vi "Configure Fixed Ref Junction [TC] Core.vi"(8 "error in (no error)":errorcluster, 10 "fixed ref junc (0.0 Celsius)":dbl format="%^.2e", 11 "IVI_DMM in":refnum<class "IVI_DMM.lvclass">) -> (0 "error out":errorcluster, 3 "IVI_DMM out":refnum<class "IVI_DMM.lvclass">)   [LabVIEW 2013, in "IVI_DMM.lvlib" / "IVI_DMM.lvclass"]
doc: "This VI configures the fixed reference junction for a thermocouple with a fixed reference junction type.\n\nThis VI affects the behavior of the instrument only when the IviDmm>Temperature Measurements>Thermocouple>Reference Junction Type [TC] property is set to IVIDMM_VAL_TEMP_REF_JUNC_FIXED.\n\nNote:\n\n(1) This VI is part of the IviDmmThermocouple [TC] extension group."
uses:
  IVI_DMM.lvclass
  IVI_DMM.lvclass/IVI_DMM.ctl
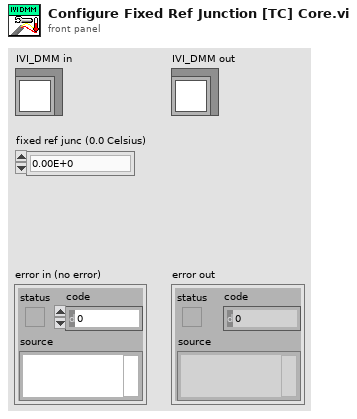
[diagram p1: front panel]
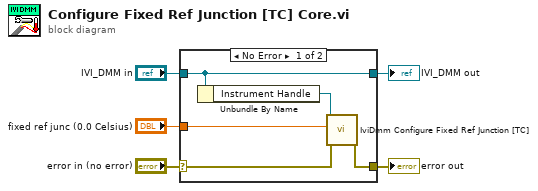
[diagram p0: block diagram]
diagram:
  n1 = case shown="No Error" "error in (no error)" {
    selector: "error in (no error)" -> [w7 w12]
    tunnel: [w9 w12] -> w4
    tunnel: [w10 w11] -> w2
    tunnel: "IVI_DMM in" -> [w10 w11]
    tunnel: "fixed ref junc (0.0 Celsius)" -> [w6 _]
    frame No Error {
      n2 = Unbundle By Name(w10) -> ("Instrument Handle"=w8:refnum<k15>)
      n3 = call <vilib>:"IviDmm Configure Fixed Ref Junction [TC].vi"("error in (no error)"=w7, "fixed ref junc (0.0 Celsius)"=w6, "instrument handle"=w8) -> ("error out"=w9:errorcluster)  [unwired: 7 in, 1 out]
    }
    frame Error {
    }
  }
  "error out" <- w4
  "IVI_DMM out" <- w2
